vi "CODMn仪器参数设置.vi"(11 "仪器参数设置":T2) -> (3 "仪器参数设置输出":T1)   [LabVIEW 2016]
uses:
  <vilib>/Utility/miscctls.llb/LVPointTypeDef.ctl
panel:
  in  "标样校准时间":timestamp
  in  "二次多项式系数":dbl
  in  "线性相关系数":dbl
  in  "测量信号值":dbl
  in  "测量检出限":dbl
  in  "曲线斜率":dbl
  in  "曲线截距":dbl
  in  "空白校准时间":timestamp
  in  "消解时长":dbl
  in  "消解温度":dbl
  in  "测量间隔":dbl
  in  "测量精度":dbl
  in  "测量量程":dbl
  in  "取消":bool
  in  "确定":bool
  # "仪器参数设置"
  # "CODMn"
  # "监测参数"
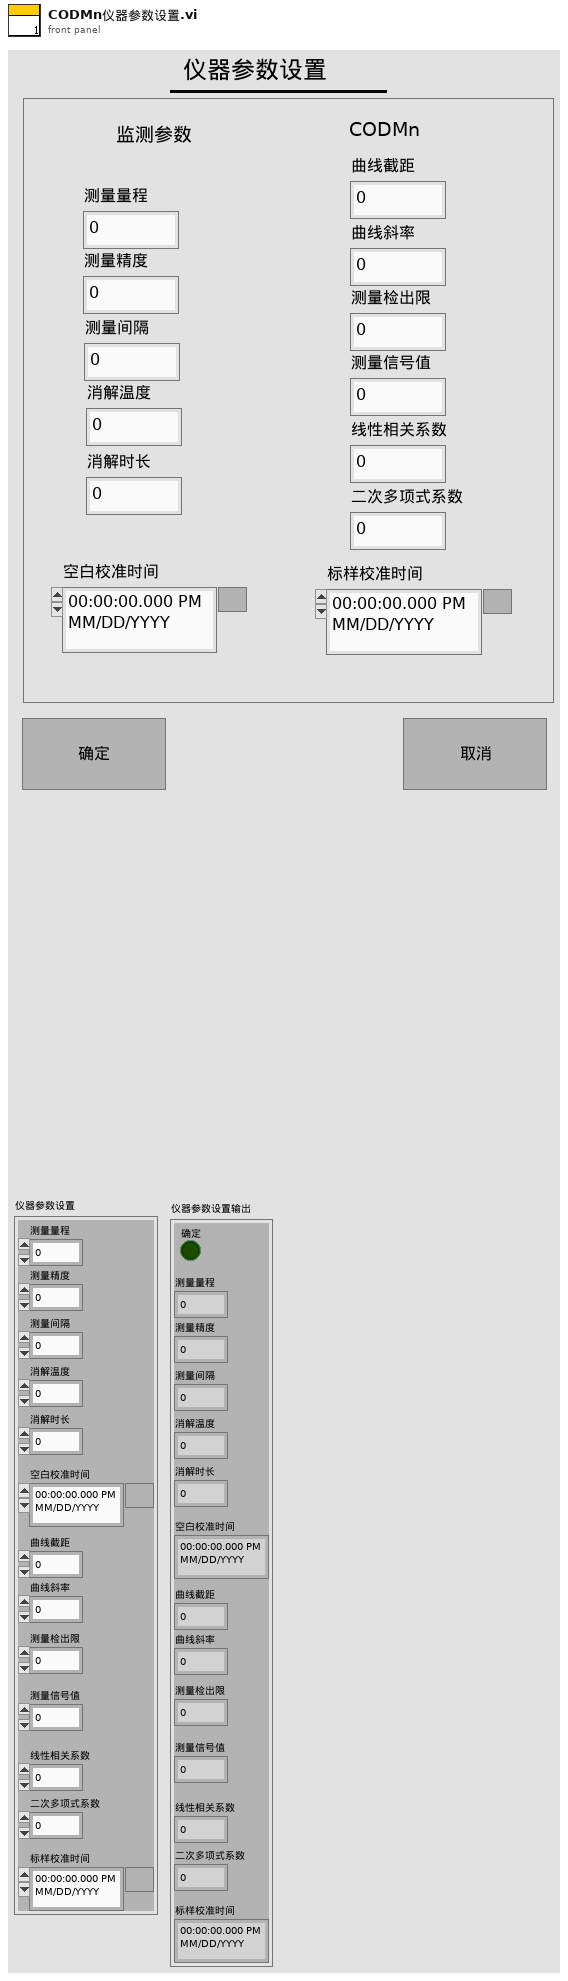
[diagram p1: front panel]
types:
  T1 = cluster{"确定":bool, "测量量程":dbl, "测量精度":dbl, "测量间隔":dbl, "消解温度":dbl, "消解时长":dbl, "空白校准时间":timestamp, "曲线截距":dbl, "曲线斜率":dbl, "测量检出限":dbl, "测量信号值":dbl, "线性相关系数":dbl, "二次多项式系数":dbl, "标样校准时间":timestamp}
  T2 = cluster{"测量量程":dbl, "测量精度":dbl, "测量间隔":dbl, "消解温度":dbl, "消解时长":dbl, "空白校准时间":timestamp, "曲线截距":dbl, "曲线斜率":dbl, "测量检出限":dbl, "测量信号值":dbl, "线性相关系数":dbl, "二次多项式系数":dbl, "标样校准时间":timestamp}
  T3 = typedef "LVPointTypeDef.ctl" = cluster{"Horizontal":i16, "Vertical":i16}
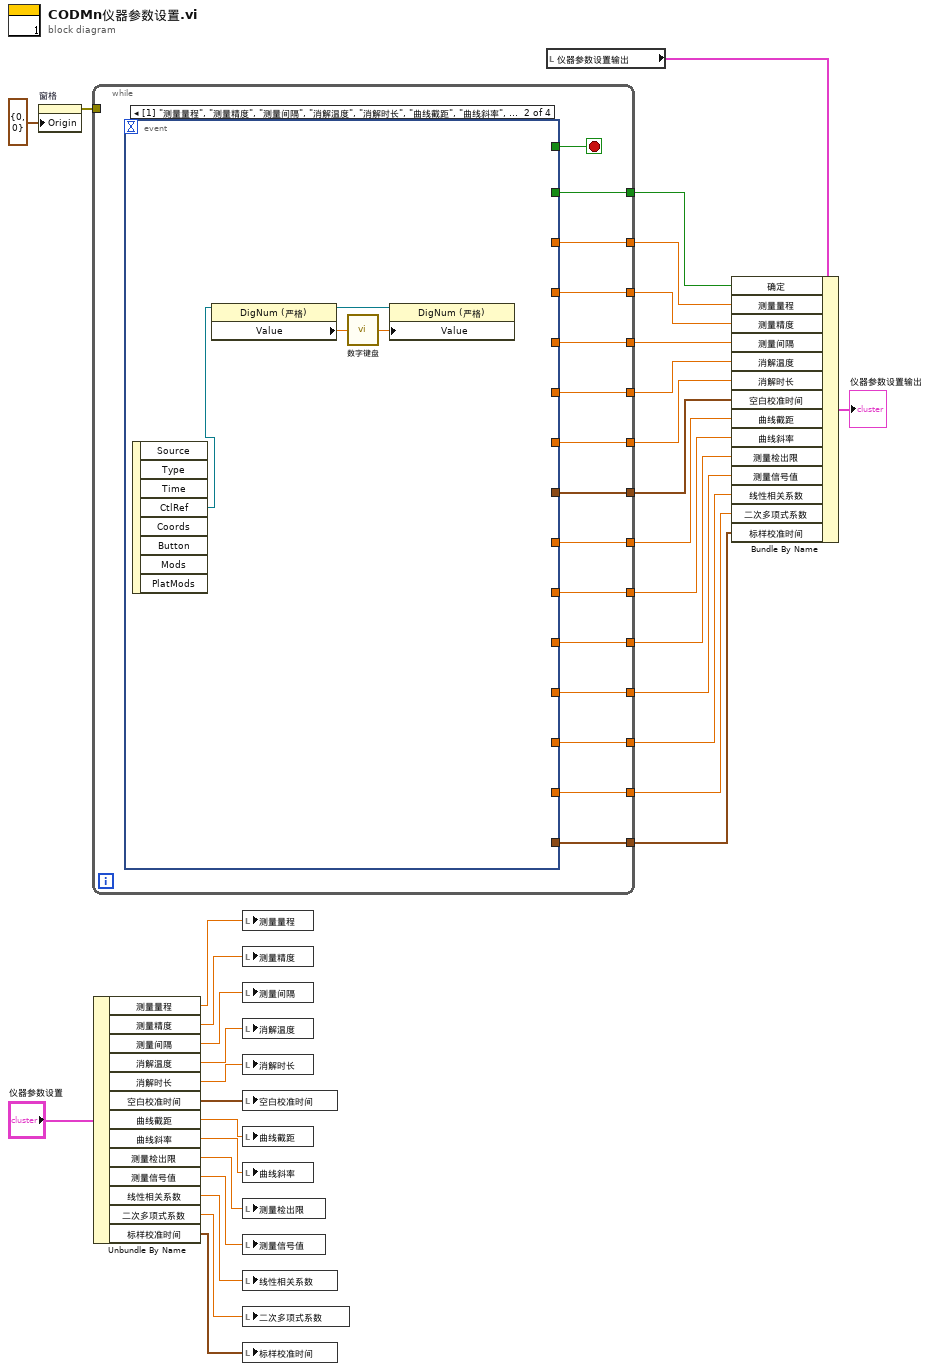
[diagram p0: block diagram]
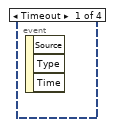
[diagram p2: hidden frame]
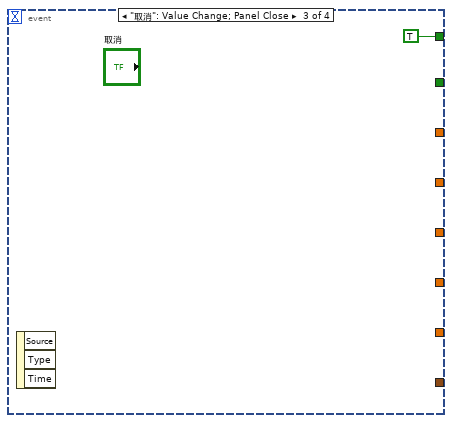
[diagram p3: hidden frame]
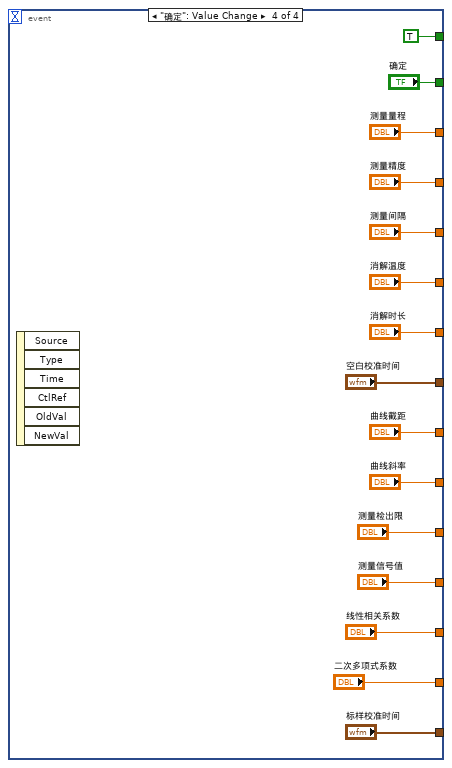
[diagram p4: hidden frame]
diagram:
  n1 = property on="窗格" class="Pane"("Origin"=T3 {"Horizontal"=0, "Vertical"=0} ("原点")) -> (error out=w31:errorcluster)  [unwired: 2 in, 1 out]
  n2 = while {
    tunnel: w31 -> [_]
    tunnel: [w46] -> w30
    tunnel: [w45] -> w26
    tunnel: [w44] -> w25
    tunnel: [w43] -> w24
    tunnel: [w42] -> w23
    tunnel: [w41] -> w22
    tunnel: [w40] -> w21
    tunnel: [w39] -> w20
    tunnel: [w38] -> w19
    tunnel: [w37] -> w18
    tunnel: [w36] -> w17
    tunnel: [w35] -> w16
    tunnel: [w34] -> w15
    tunnel: [w33] -> w14
    stop <- w47 stop-if-true
    n3 = event shown="[1] \"测量量程\", \"测量精度\", \"测量间隔\", \"消解温度\", \"消解时长\", \"曲线截距\", \"曲线斜率\", \"测量检出限\", \"测量信号值\", \"线性相关系数\", \"二次多项式系数\": 鼠标按下" {
      selector: _ -> [_ _ _ _]
      dyn-events: _ -> [_ _ _ _]
      timeout: _ -> [_ _ _ _]
      tunnel: [_ _ TRUE TRUE] -> w47
      tunnel: [_ _ _ "确定"] -> w46
      tunnel: [_ _ _ "标样校准时间"] -> w45
      tunnel: [_ _ _ "二次多项式系数"] -> w44
      tunnel: [_ _ _ "线性相关系数"] -> w43
      tunnel: [_ _ _ "测量信号值"] -> w42
      tunnel: [_ _ _ "测量检出限"] -> w41
      tunnel: [_ _ _ "曲线斜率"] -> w40
      tunnel: [_ _ _ "曲线截距"] -> w39
      tunnel: [_ _ _ "空白校准时间"] -> w38
      tunnel: [_ _ _ "消解时长"] -> w37
      tunnel: [_ _ _ "消解温度"] -> w36
      tunnel: [_ _ _ "测量间隔"] -> w35
      tunnel: [_ _ _ "测量精度"] -> w34
      tunnel: [_ _ _ "测量量程"] -> w33
      event Timeout {
        n4 = event-data() -> ()  [unwired: 1 in, 3 out]
      }
      event "测量量程", "测量精度", "测量间隔", "消解温度", "消解时长", "曲线截距", "曲线斜率", "测量检出限", "测量信号值", "线性相关系数", "二次多项式系数": Mouse Down {
        n5 = event-data() -> ("CtlRef"=w48:refnum<vi>)  [unwired: 1 in, 7 out]
        n6 = property class="DigNum (严格)"(reference=w48) -> (reference out=w50:refnum<vi>, "Value"=w51:dbl)  [unwired: 1 in, 1 out]
        n7 = call "数字键盘.vi"("OldNumber"=w51) -> ("NewNumber"=w49:sgl)
        n8 = property class="DigNum (严格)"(reference=w50, "Value"=w49) -> ()  [unwired: 1 in, 2 out]
      }
      event "取消": Value Change; Panel Close {
        n9 = event-data() -> ()  [unwired: 1 in, 3 out]
      }
      event "确定": Value Change {
        n10 = event-data() -> ()  [unwired: 1 in, 6 out]
      }
    }
  }
  n11 = Unbundle By Name("仪器参数设置") -> ("测量量程"=w13:dbl, "测量精度"=w12:dbl, "测量间隔"=w11:dbl, "消解温度"=w10:dbl, "消解时长"=w9:dbl, "空白校准时间"=w8:timestamp, "曲线截距"=w7:dbl, "曲线斜率"=w6:dbl, "测量检出限"=w5:dbl, "测量信号值"=w4:dbl, "线性相关系数"=w3:dbl, "二次多项式系数"=w2:dbl, "标样校准时间"=w1:timestamp)
  n12 = local write "测量量程"(w13) -> ()
  n13 = local write "测量精度"(w12) -> ()
  n14 = local write "测量间隔"(w11) -> ()
  n15 = local write "消解温度"(w10) -> ()
  n16 = local write "消解时长"(w9) -> ()
  n17 = local write "空白校准时间"(w8) -> ()
  n18 = local write "曲线截距"(w7) -> ()
  n19 = local write "曲线斜率"(w6) -> ()
  n20 = local write "测量检出限"(w5) -> ()
  n21 = local write "测量信号值"(w4) -> ()
  n22 = local write "线性相关系数"(w3) -> ()
  n23 = local write "二次多项式系数"(w2) -> ()
  n24 = local write "标样校准时间"(w1) -> ()
  n25 = local read "仪器参数设置输出"() -> (w28:T1)
  n26 = Bundle By Name(cluster=w28, "确定"=w30, "测量量程"=w14, "测量精度"=w15, "测量间隔"=w16, "消解温度"=w17, "消解时长"=w18, "空白校准时间"=w19, "曲线截距"=w20, "曲线斜率"=w21, "测量检出限"=w22, "测量信号值"=w23, "线性相关系数"=w24, "二次多项式系数"=w25, "标样校准时间"=w26) -> (→"仪器参数设置输出":T1)
